vi "Equation.vi"(7 "10bit":bool=TRUE, 8 "error in (no error)":errorcluster, 10 "Value":u16, 11 "Sensor Type":T1) -> (0 "error out":errorcluster, 3 "Result":dbl)   [LabVIEW 2019]
uses:
  Sensor.ctl
  <vilib>/express/express arith-compare/Formula/XNode/ExpressFormulaBlockNode.xnode
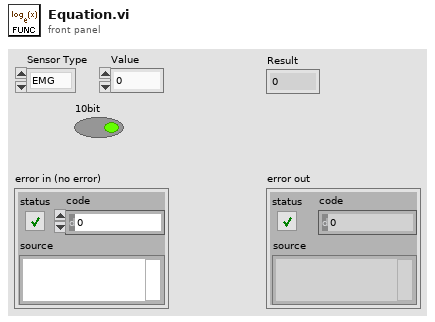
[diagram p1: front panel]
types:
  T1 = typedef "Sensor.ctl" = enum16{"EMG", "ECG", "EEG", "EDA", "ACC", "LUX"}
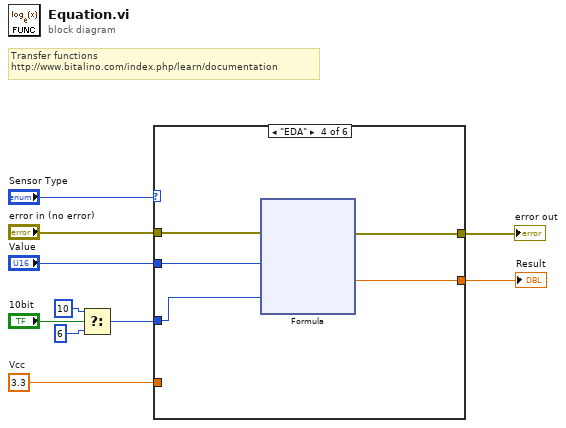
[diagram p0: block diagram]
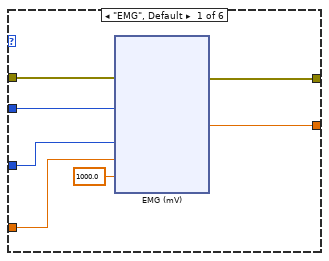
[diagram p2: hidden frame]
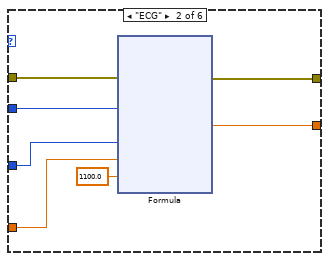
[diagram p3: hidden frame]
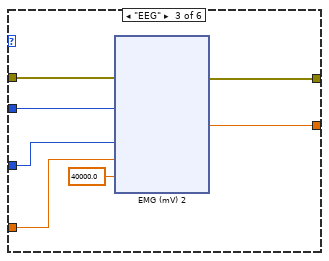
[diagram p4: hidden frame]
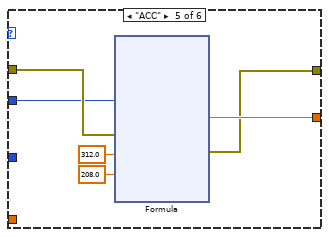
[diagram p5: hidden frame]
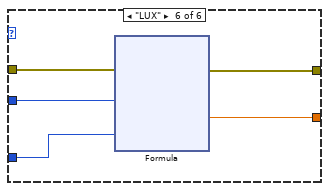
[diagram p6: hidden frame]
diagram:
  w1 = 3.3  # Vcc
  # "Transfer functions\nhttp://www.bitalino.com/index.php/learn/documentation"
  n1 = Select(t=10, s="10bit", f=6) -> (s? t:f=w5:i32)
  n2 = case shown="\"EDA\"" "Sensor Type" {
    tunnel: "Value" -> [w15 w38 w59 w77 w89 w110]
    tunnel: w5 -> [w16 w37 w55 w78 _ w111]
    tunnel: [w17 w36 w56 w76 w93 w109] -> w4
    tunnel: [w13 w35 w57 w75 w92 w107] -> w3
    tunnel: "error in (no error)" -> [w14 w34 w58 w74 w94 w108]
    tunnel: w1 -> [w11 w33 w54 _ _ _]
    frame "EMG", Default {
      n3 = xnode ("EMG (mV)")("EMG"=w15, "n"=w16, "Vcc"=w11, "Gain"=1000.0, "error in (no error)"=w14) -> ("Result"=w17:dbl, "error out"=w13:errorcluster)
    }
    frame "ECG" {
      n4 = xnode "Formula"("ECG"=w38, "n"=w37, "Vcc"=w33, "Gain"=1100.0, "error in (no error)"=w34) -> ("Result"=w36:dbl, "error out"=w35:errorcluster)
    }
    frame "EEG" {
      n5 = xnode ("EMG (mV) 2")("EEG"=w59, "n"=w55, "Vcc"=w54, "Gain"=40000.0, "error in (no error)"=w58) -> ("Result"=w56:dbl, "error out"=w57:errorcluster)
    }
    frame "EDA" {
      n6 = xnode "Formula"("EDA"=w77, "n"=w78, "error in (no error)"=w74) -> ("Result"=w76:dbl, "error out"=w75:errorcluster)
    }
    frame "ACC" {
      n7 = xnode "Formula"("ACC"=w89, "error in (no error)"=w94, "CM"=312.0, "Cm"=208.0) -> ("Result"=w93:dbl, "error out"=w92:errorcluster)
    }
    frame "LUX" {
      n8 = xnode "Formula"("LUX"=w110, "n"=w111, "error in (no error)"=w108) -> ("Result"=w109:dbl, "error out"=w107:errorcluster)
    }
  }
  "Result" <- w4
  "error out" <- w3
